vi "LUCS001RT_GPS_GPGGAGetTimeOfFix.vi"(2 "String:CurrentPosition.TimeOfFix":string="170834") -> (6 "CurrentPosition.TimeOfFix":u32 format="%<%H:%M:%S>t")   [LabVIEW 2020]
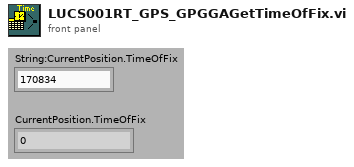
[diagram p1: front panel]
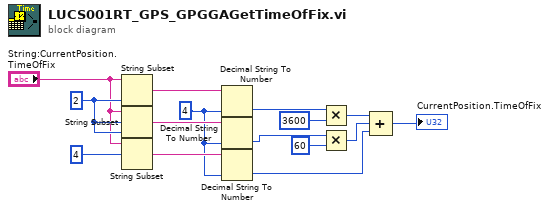
[diagram p0: block diagram]
diagram:
  w10 = 4 ("offset (0)")
  w15 = 2 ("length (rest)")
  n1 = String Subset(string="String:CurrentPosition.TimeOfFix", length (rest)=w15) -> (substring=w13:string)  [unwired: 1 in]
  n2 = String Subset(string="String:CurrentPosition.TimeOfFix", offset (0)=w15, length (rest)=w15) -> (substring=w12:string)
  n3 = String Subset(string="String:CurrentPosition.TimeOfFix", offset (0)=4) -> (substring=w11:string)  [unwired: 1 in]
  n4 = Decimal String To Number(string=w13, default (0L)=w10) -> (number=w7:i32)  [unwired: 1 in, 1 out]
  n5 = Decimal String To Number(string=w12, default (0L)=w10) -> (number=w5:i32)  [unwired: 1 in, 1 out]
  n6 = Decimal String To Number(string=w11, default (0L)=w10) -> (number=w2:i32)  [unwired: 1 in, 1 out]
  n7 = Multiply(x=w7, y=3600) -> (x*y=w8:i32)
  n8 = Multiply(x=w5, y=60) -> (x*y=w3:i32)
  n9 = Compound Arithmetic op=ADD(w8, w3, w2) -> (→"CurrentPosition.TimeOfFix":i32)
